vi "widmo_mocy_SubVi.vi"(11 "signal in":waveform(dbl)) -> (3 "widmo mocy":waveform(dbl)(graph))   [LabVIEW 2025]
uses:
  <vilib>/Analysis/NI_AALPro.lvlib
  <vilib>/Analysis/2dsp.llb/Real FFT.vi
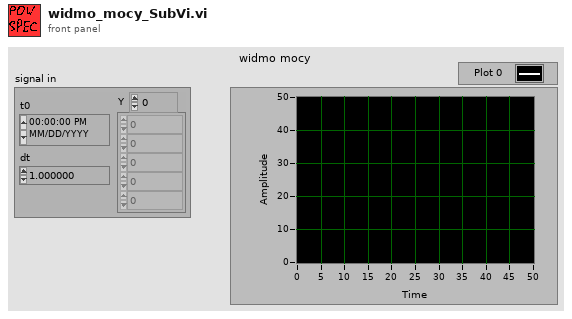
[diagram p1: front panel]
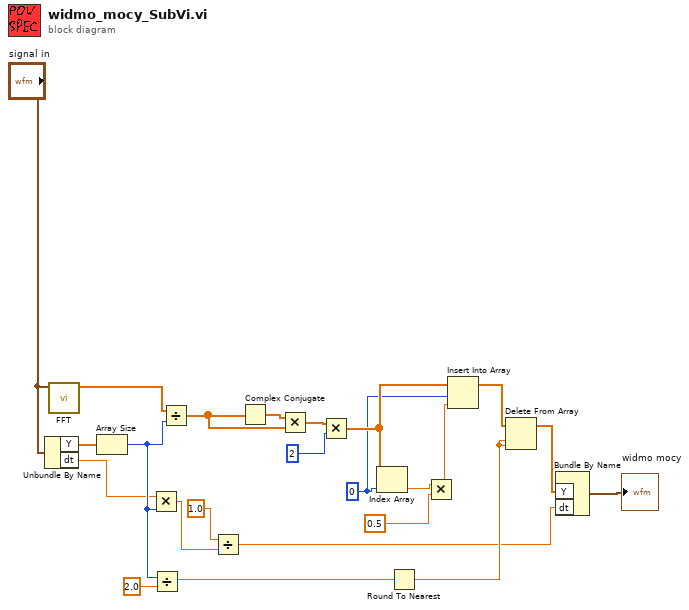
[diagram p0: block diagram]
diagram:
  w8 = 0 ("index")
  n1 = Unbundle By Name("signal in") -> ("Y"=w2:dbl[], "dt"=w16:dbl)
  n2 = call-poly <vilib>:"FFT.vi"("X"="signal in") -> ("FFT {X}"=w3:cdb[])  [unwired: 9 in, 1 out]
  n3 = Array Size(array=w2) -> (size(s)=w21:i32)
  n4 = Multiply(x=w16, y=w21) -> (x*y=w17:dbl)
  n5 = Divide(x=w21, y=2.0) -> (x/y=w22:dbl)
  n6 = Divide(x=w3, y=w21) -> (x/y=w5:cdb[])
  n7 = Divide(x=1.0, y=w17) -> (x/y=w19:dbl)
  n8 = Complex Conjugate(1:w5) -> (0:w4:cdb[])
  n9 = Multiply(x=w4, y=w5) -> (x*y=w6:cdb[])
  n10 = Multiply(x=w6, y=2 ("index")) -> (x*y=w9:cdb[])
  n11 = Index Array(array=w9, index=w8) -> (element=w10:cdb)
  n12 = Round To Nearest(number=w22) -> (nearest integer value=w23:dbl)
  n13 = Multiply(x=w10, y=0.5 ("index")) -> (x*y=w12:cdb)
  n14 = Insert Into Array(array=w9, index=w8, new element=w12) -> (w13:cdb[])
  n15 = Delete From Array(array=w13, length=w23, index=w23) -> (array with subset deleted=w14:cdb[])  [unwired: 1 out]
  n16 = Bundle By Name("Y"=w14, "dt"=w19) -> (→"widmo mocy":waveform(cdb))  [unwired: 1 in]
